vi "Reverse Find.vi"(7 "Character":string, 11 "String":string) -> (3 "Position":i32)   [LabVIEW 2018, in "Toolkit.lvlib" / "Parser.lvclass"]
uses:
  Parser.lvclass
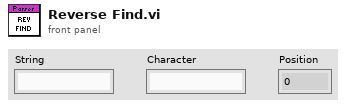
[diagram p1: front panel]
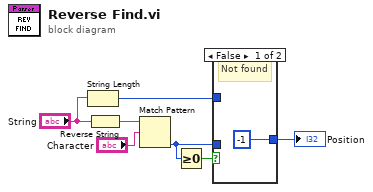
[diagram p0: block diagram]
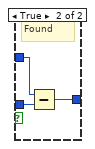
[diagram p2: hidden frame]
diagram:
  n1 = String Length(string="String") -> (length=w3:i32)
  n2 = Reverse String(1:"String") -> (0:w2:string)
  n3 = Match Pattern(string=w2, regular expression="Character") -> (offset past match=w6:i32)  [unwired: 1 in, 3 out]
  n4 = Greater Or Equal To 0?(x=w6) -> (x >= 0?=w4:bool)
  n5 = case shown="False" w4 {
    tunnel: w3 -> [_ w11]
    tunnel: w6 -> [_ w10]
    tunnel: [-1 w9] -> w7
    frame False {
      # "Not found"
    }
    frame True {
      # "Found"
      n6 = Subtract(x=w11, y=w10) -> (x-y=w9:i32)
    }
  }
  "Position" <- w7
